vi "jMsg_TCPClient_Message_Send (create).vi"(8 "error in (no error)":errorcluster, 11 "Packet":refnum<class "TCPPacket.lvclass">) -> (0 "error out":errorcluster, 3 "jMsg_TCPClient_Message_Send":refnum<class "jMsg_TCPClient_Message_Send.lvclass">)   [LabVIEW 2019, in "jMsg_TCPClient_Message_Send.lvclass"]
doc: "This VI is used to create the jMsg\n\n\nJSMA Message Wizard 0.2.0.5\nRob Humfeld - Jet Engineering\nCopyright (c) 2020, Jet Engineering"
uses:
  jMsg_TCPClient_Message_Send.lvclass
  C:/Program Files/National Instruments/LabVIEW 2019/user.lib/Jet Engineering/JSMA/Libraries/jMsg Class/jMsg.lvclass
  <userlib>/Jet Engineering/JSMA/Libraries/jMsg Class/jMsg.lvclass/jMsg.ctl
  <userlib>/Jet Engineering/JSMA/Libraries/Shared/JSMA_GetClassName.vi
  <vilib>/Utility/LVClass/Get LV Class Path.vi
  <userlib>/Jet Engineering/JSMA/Libraries/jMsg Class/jMsg.lvclass
  TCPPacket/TCPPacket.lvclass
panel:
  in  "jMsg_TCPClient_Message_Send":refnum<class "jMsg_TCPClient_Message_Send.lvclass">
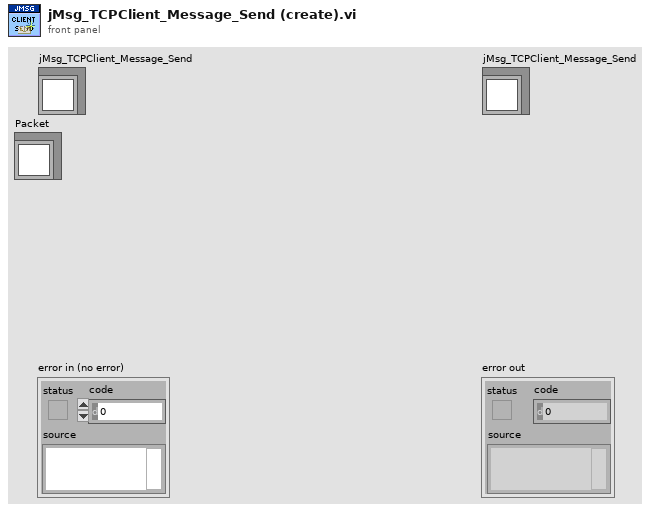
[diagram p1: front panel]
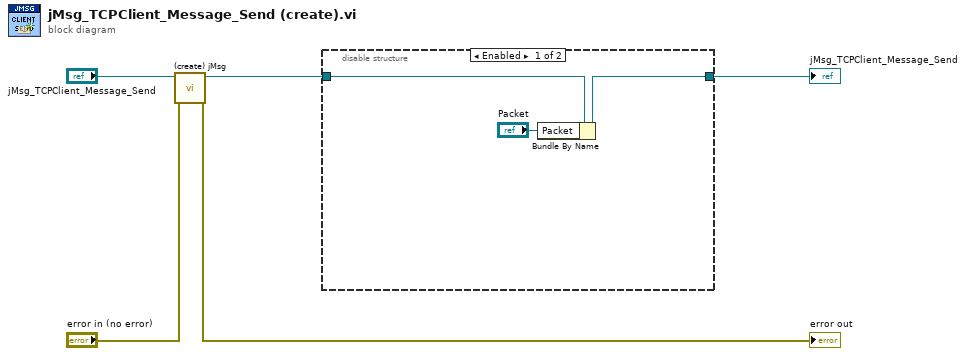
[diagram p0: block diagram]
diagram:
  n1 = call <userlib>:"(create) jMsg.vi"("error in (no error)"="error in (no error)", "jMsg in"="jMsg_TCPClient_Message_Send") -> ("error out"=→"error out":errorcluster, "jMsg out"=w1:refnum<class "jMsg_TCPClient_Message_Send.lvclass">)  [unwired: 8 in]
  n2 = disable-structure shown="Enabled" {
    disable-tunnel: w1 -> [w8 w9]
    disable-tunnel: [w7 w9] -> w5
    frame Enabled {
      n3 = Bundle By Name(cluster=w8, "Packet"="Packet") -> (w7:refnum<class "jMsg_TCPClient_Message_Send.lvclass">)
    }
    frame Disabled {
    }
  }
  "jMsg_TCPClient_Message_Send" <- w5
